vi "LINC Daemon Client.vi"(6 "instance":i32, 7 "timeout ms (1000)":i32=1000, 8 "port config":T1, 9 "port":u16, 10 "address":string, 11 "LINC session":refnum<class "LINC.lvclass">) -> ()   [LabVIEW 2018, in "STEPkgDriver_LINC.lvlib" / "LINC.lvclass"]
uses:
  LINC.lvclass
  STEPkgDriver_LINC.lvlib
  LINC Global Mode.ctl
  LINC Global Config Mode.ctl
  LINC Global Session Mode.ctl
  LINC Global Handshake Mode.ctl
  LINC Handshake Internal.ctl
  LINC Command Origin.ctl
  LINC Handshake.ctl
  LINC Daemon Manager Mode.ctl
  LINC Port Config.ctl
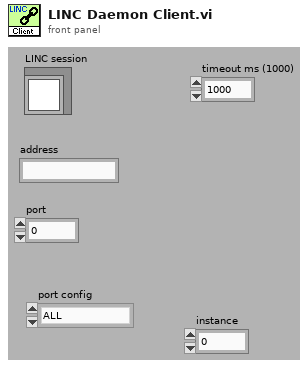
[diagram p1: front panel]
types:
  T1 = typedef "STEPkgDriver_LINC.lvlib/LINC Port Config.ctl" = enum16{"ALL", "CMD_ALL", "TLM_ALL", "TLM_BASIC"}
  T2 = typedef "STEPkgDriver_LINC.lvlib/LINC Global Config Mode.ctl" = enum16{"INIT", "CLEAR", "SET_CMD_CB", "SET_TLM_CB", "SET_CMD_FIELDS", "SET_TLM_FIELDS", "SET_ID", "GET_CONFIG"}
  T3 = typedef "STEPkgDriver_LINC.lvlib/LINC Global Mode.ctl" = enum16{"INIT", "CLEAR", "ADD_PKT_HDR", "ADD_PKT", "GET_PKT_NAMES", "GET_PKT_DESC", "GET_PKT_HDR", "GET_PKT", "SET_PKT", "SET_DATA", "SIM_EN", "SIM_DS"}
  T4 = typedef "STEPkgDriver_LINC.lvlib/LINC Config.ctl" = cluster{"cmd callback":refnum<vi>, "tlm callback":refnum<vi>, "cmd ID bitoffset":i32, "cmd ID bitsize":i32, "cmd IDs":i32[], "tlm ID bitoffset":i32, "tlm ID bitsize":i32, "tlm IDs":i32[], "cmd header fields":i32, "tlm header fields":i32, "tlm header size":i32}
  T5 = typedef "STEPkgDriver_LINC.lvlib/LINC Daemon Manager Mode.ctl" = enum16{"INIT", "CLEAR", "GET"}
  T6 = typedef "STEPkgDriver_LINC.lvlib/LINC Global Session Mode.ctl" = enum16{"INIT", "CLEAR", "ADD_SESSION", "SET_CONNECTION", "SET_LISTENER", "SET_REFERENCE", "GET_SESSION"}
  T7 = cluster{"binary value (F)":bool, "include unit (F)":bool}
  T8 = typedef "STEPkgDriver_LINC.lvlib/LINC Handshake Internal.ctl" = cluster{"error":errorcluster, "command data":string}
  T9 = typedef "STEPkgDriver_LINC.lvlib/LINC Global Handshake Mode.ctl" = enum16{"INIT", "CLEAR", "ADD_COMMAND", "RMV_COMMAND", "CLR_HANDSHAKE", "SET_HANDSHAKE", "GET_HANDSHAKE"}
  T10 = typedef "STEPkgDriver_LINC.lvlib/LINC Handshake.ctl" = cluster{"ORIGIN":T11, "STATUS":bool, "CODE":i32, "TIME_SECONDS":u32, "TIME_MICROSECONDS":u32, "DATA":string}
  T11 = typedef "STEPkgDriver_LINC.lvlib/LINC Command Origin.ctl" = enum8{"RMT", "LCL"}
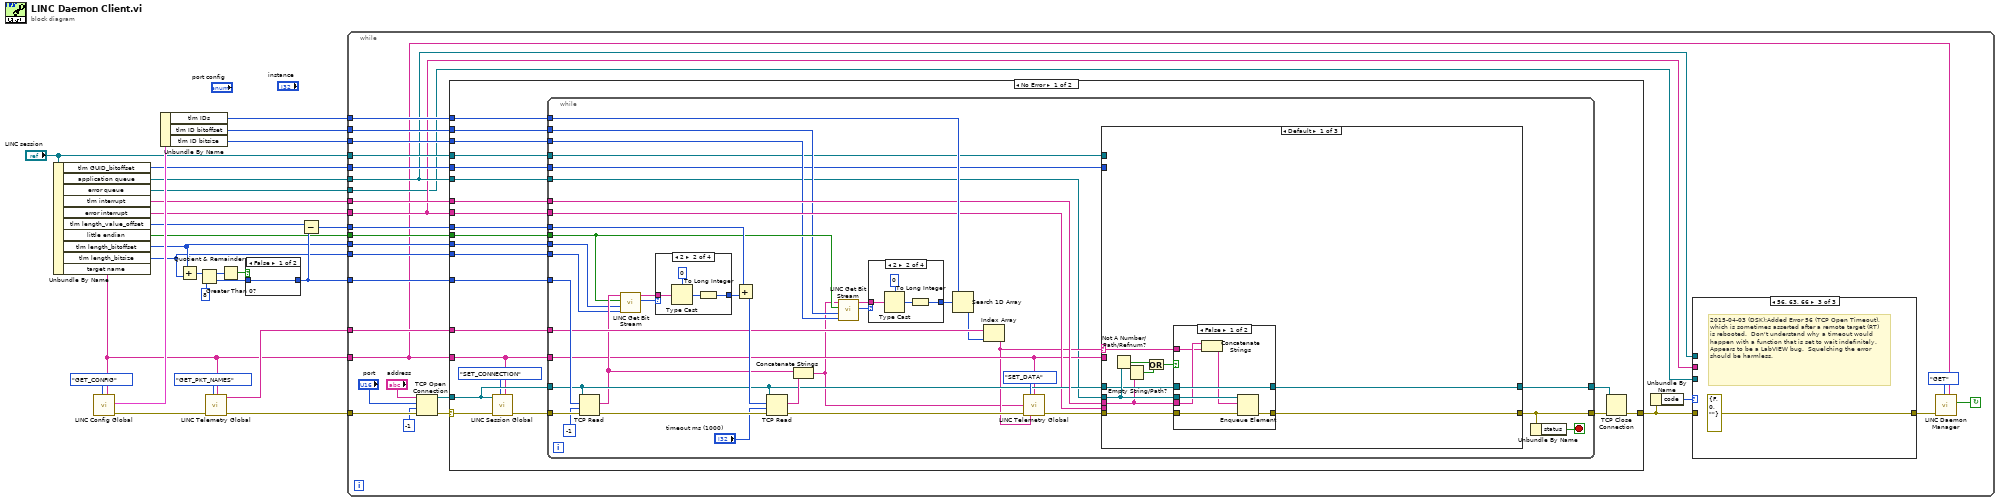
[diagram p0: block diagram]
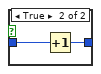
[diagram p2: hidden frame]
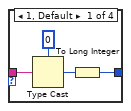
[diagram p3: hidden frame]
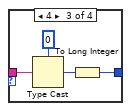
[diagram p4: hidden frame]
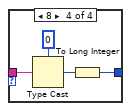
[diagram p5: hidden frame]
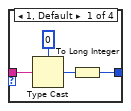
[diagram p6: hidden frame]
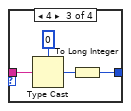
[diagram p7: hidden frame]
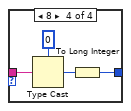
[diagram p8: hidden frame]
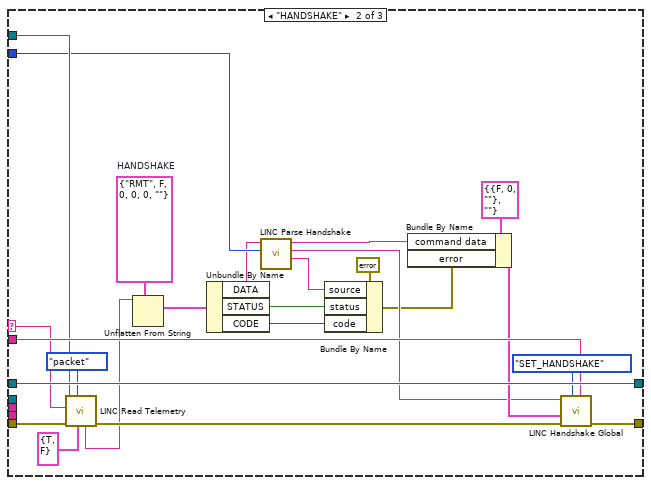
[diagram p10: hidden frame]
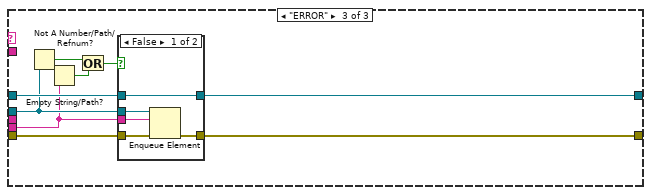
[diagram p11: hidden frame]
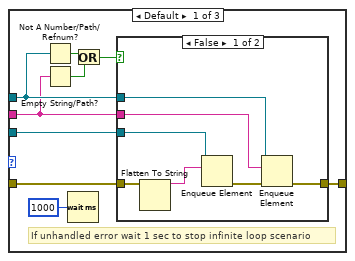
[diagram p14: hidden frame]
diagram:
  n1 = Unbundle By Name("LINC session") -> ("tlm GUID_bitoffset"=w3:i32, "application queue"=w8:refnum<queue>, "error queue"=w1:refnum<queue>, "tlm interrupt"=w9:string, "error interrupt"=w7:string, "tlm length_value_offset"=w10:i32, "little endian"=w6:bool, "tlm length_bitoffset"=w5:i32, "tlm length_bitsize"=w4:i32, "target name"=w11:string)
  n2 = call "LINC Config Global.vi"("target name"=w11, "mode"=LINC_Global_Config_Mode."GET_CONFIG") -> ("error out"=w26:errorcluster, "config out"=w24:T4)  [unwired: 8 in]
  n3 = Unbundle By Name(w24) -> ("tlm IDs"=w23:i32[], "tlm ID bitoffset"=w22:i32, "tlm ID bitsize"=w21:i32)
  n4 = Add(x=w5, y=w4) -> (x+y=w15:i32)
  n5 = Quotient & Remainder(x=w15, y=8) -> (x-y*floor(x/y)=w17:i32, floor(x/y)=w19:i32)
  n6 = call "LINC Telemetry Global.vi"("mode"=LINC_Global_Mode."GET_PKT_NAMES", "target name"=w11, "error in (no error)"=w26) -> ("values out"=w20:string[], "error out"=w25:errorcluster)  [unwired: 8 in, 3 out]
  n7 = Greater Than 0?(x=w17) -> (x > 0?=w18:bool)
  n8 = case shown="False" w18 {
    tunnel: w19 -> [w28 w30]
    tunnel: [w28 w29] -> w13
    frame False {
    }
    frame True {
      n9 = Increment(x=w30) -> (x+1=w29:i32)
    }
  }
  n10 = Subtract(x=w10, y=w13) -> (x-y=w14:i32)
  n11 = while {
    tunnel: w11 -> [w32]
    tunnel: w25 -> [w55]
    tunnel: w23 -> [w54]
    tunnel: w22 -> [w53]
    tunnel: w21 -> [w52]
    tunnel: w20 -> [w51]
    tunnel: w14 -> [w50]
    tunnel: w13 -> [w49]
    tunnel: w9 -> [w48]
    tunnel: w8 -> [w38]
    tunnel: w7 -> [w37]
    tunnel: w6 -> [w45]
    tunnel: w5 -> [w44]
    tunnel: w4 -> [w43]
    tunnel: w3 -> [w42]
    tunnel: "LINC session" -> [w41]
    tunnel: w1 -> [w36]
    stop <- w33 continue-if-true
    n12 = TCP Open Connection(address="address", remote port or service name="port", timeout ms (60000)=-1, error in (no error)=w55) -> (connection ID=w46:refnum<k5>, error out=w31:errorcluster)  [unwired: 1 in]
    n13 = case shown="No Error" w31 {
      selector: w31 -> [w58 w209]
      tunnel: w54 -> [w78 _]
      tunnel: w53 -> [w77 _]
      tunnel: w52 -> [w76 _]
      tunnel: w51 -> [w75 _]
      tunnel: w50 -> [w72 _]
      tunnel: w49 -> [w71 _]
      tunnel: w48 -> [w70 _]
      tunnel: w46 -> [w69 _]
      tunnel: w45 -> [w67 _]
      tunnel: w44 -> [w66 _]
      tunnel: w43 -> [w65 _]
      tunnel: w42 -> [w64 _]
      tunnel: w41 -> [w63 _]
      tunnel: [w62 w209] -> w39
      tunnel: w38 -> [w61 _]
      tunnel: w37 -> [w60 _]
      tunnel: w32 -> [w59 _]
      frame No Error {
        n14 = call "LINC Session Global.vi"("target name"=w59, "mode"=LINC_Global_Session_Mode."SET_CONNECTION", "error in (no error)"=w58, "connection in"=w69) -> ("error out"=w79:errorcluster)  [unwired: 3 in, 4 out]
        n15 = while {
          tunnel: w79 -> [w117]
          tunnel: w69 -> [w101]
          tunnel: [w103] -> w74
          tunnel: [w100] -> w73
          tunnel: w71 -> [w112]
          tunnel: w72 -> [w111]
          tunnel: w76 -> [w88]
          tunnel: w77 -> [w89]
          tunnel: w78 -> [w108]
          tunnel: w75 -> [w109]
          tunnel: w59 -> [w86]
          tunnel: w70 -> [w102]
          tunnel: w61 -> [w81]
          tunnel: w60 -> [w99]
          tunnel: w67 -> [w90]
          tunnel: w66 -> [w94]
          tunnel: w65 -> [w93]
          tunnel: w64 -> [w84]
          tunnel: w63 -> [w82]
          stop <- w115 stop-if-true
          n16 = TCP Read(connection ID=w101, bytes to read=w112, error in (no error)=w117, 9:-1 ("timeout ms (25000)")) -> (data out=w95:string, error out=w114:errorcluster)  [unwired: 2 out]
          n17 = call "LINC Get Bit Stream.vi"("bit size"=w93, "bit offset"=w94, "little endian"=w90, "data in"=w95) -> ("bytes"=w98:i32, "data out"=w97:string)  [unwired: 6 in]
          n18 = case shown="2" w98 {
            tunnel: w97 -> [w137 w141 w145 w149]
            tunnel: [w134 w138 w142 w146] -> w96
            frame 1, Default {
              n19 = Type Cast(type=u8 0, x=w137) -> (*(type *) &x=w135:u8)
              n20 = To Long Integer(number=w135) -> (32bit integer=w134:i32)
            }
            frame 2 {
              n21 = Type Cast(type=u16 0, x=w141) -> (*(type *) &x=w139:u16)
              n22 = To Long Integer(number=w139) -> (32bit integer=w138:i32)
            }
            frame 4 {
              n23 = Type Cast(type=u32 0, x=w145) -> (*(type *) &x=w143:u32)
              n24 = To Long Integer(number=w143) -> (32bit integer=w142:i32)
            }
            frame 8 {
              n25 = Type Cast(type=u64 0, x=w149) -> (*(type *) &x=w147:u64)
              n26 = To Long Integer(number=w147) -> (32bit integer=w146:i32)
            }
          }
          n27 = Add(x=w111, y=w96) -> (x+y=w110:i32)
          n28 = TCP Read(connection ID=w101, bytes to read=w110, error in (no error)=w114, 9:"timeout ms (1000)") -> (data out=w113:string, error out=w105:errorcluster)  [unwired: 2 out]
          n29 = Concatenate Strings(w95, w113) -> (w83:string)
          n30 = call "LINC Get Bit Stream.vi"("bit size"=w88, "bit offset"=w89, "little endian"=w90, "data in"=w83) -> ("bytes"=w91:i32, "data out"=w92:string)  [unwired: 6 in]
          n31 = case shown="2" w91 {
            tunnel: w92 -> [w121 w125 w129 w133]
            tunnel: [w118 w122 w126 w130] -> w87
            frame 1, Default {
              n32 = Type Cast(type=u8 0, x=w121) -> (*(type *) &x=w119:u8)
              n33 = To Long Integer(number=w119) -> (32bit integer=w118:i32)
            }
            frame 2 {
              n34 = Type Cast(type=u16 0, x=w125) -> (*(type *) &x=w123:u16)
              n35 = To Long Integer(number=w123) -> (32bit integer=w122:i32)
            }
            frame 4 {
              n36 = Type Cast(type=u32 0, x=w129) -> (*(type *) &x=w127:u32)
              n37 = To Long Integer(number=w127) -> (32bit integer=w126:i32)
            }
            frame 8 {
              n38 = Type Cast(type=u64 0, x=w133) -> (*(type *) &x=w131:u64)
              n39 = To Long Integer(number=w131) -> (32bit integer=w130:i32)
            }
          }
          n40 = Search 1D Array(1D array=w108, element=w87) -> (index of element=w107:i32)  [unwired: 1 in]
          n41 = Index Array(array=w109, index=w107) -> (element=w85:string)
          n42 = call "LINC Telemetry Global.vi"("mode"=LINC_Global_Mode."SET_DATA", "target name"=w86, "data in"=w83, "error in (no error)"=w105, "packet name"=w85) -> ("error out"=w104:errorcluster)  [unwired: 6 in, 4 out]
          n43 = case shown="Default" w85 {
            selector: w85 -> [w150 w186 _]
            tunnel: w104 -> [w159 w187 w201]
            tunnel: [w158 w190 w200] -> w103
            tunnel: w102 -> [w154 _ _]
            tunnel: w81 -> [w157 _ w195]
            tunnel: w101 -> [w156 w192 w199]
            tunnel: [w155 w192 w198] -> w100
            tunnel: w99 -> [_ _ w194]
            tunnel: w86 -> [_ w189 _]
            tunnel: w84 -> [_ w183 _]
            tunnel: w82 -> [_ w184 _]
            frame Default {
              n44 = Not A Number/Path/Refnum?(number/path/refnum=w157) -> (NaN/Path/Refnum?=w153:bool)
              n45 = Empty String/Path?(string/path=w154) -> (empty?=w152:bool)
              n46 = Or(x=w153, y=w152) -> (x .or. y?=w151:bool)
              n47 = case shown="False" w151 {
                tunnel: w159 -> [w166 w168]
                tunnel: [w165 w168] -> w158
                tunnel: w157 -> [w164 _]
                tunnel: w154 -> [w161 _]
                tunnel: w156 -> [w163 w167]
                tunnel: [w163 w167] -> w155
                tunnel: w150 -> [w160 _]
                frame False {
                  n48 = Concatenate Strings(w161, w160) -> (w162:string)
                  n49 = Enqueue Element(queue=w164, element=w162, error in (no error)=w166) -> (error out=w165:errorcluster)  [unwired: 1 in, 2 out]
                }
                frame True {
                }
              }
            }
            frame "HANDSHAKE" {
              w180 = T10 {"ORIGIN"=enum."RMT", "STATUS"=FALSE, "CODE"=0, "TIME_SECONDS"=0, "TIME_MICROSECONDS"=0, "DATA"=""}  # HANDSHAKE
              n50 = call "LINC Read Telemetry.vi"("options"=T7 {"binary value (F)"=TRUE, "include unit (F)"=FALSE}, "mode (single)"=enum16{"single", "packet", "all"}."packet", "error in (no error)"=w187, "packet name"=w186, "LINC session"=w184) -> ("error out"=w185:errorcluster, "flattened data"=w179:string)  [unwired: 2 in, 3 out]
              n51 = Unflatten From String(type=w180, binary string=w179) -> (value=w178:T10)  [unwired: 3 in, 2 out]
              n52 = Unbundle By Name(w178) -> ("DATA"=w177:string, "STATUS"=w174:bool, "CODE"=w173:i32)
              n53 = call "LINC Parse Handshake.vi"("GUID bitoffset"=w183, "command packet"=w177) -> ("error source"=w169:string, "GUID"=w172:string, "command data"=w170:string)  [unwired: 7 in]
              n54 = Bundle By Name(cluster=errorcluster {"status"=FALSE, "code"=0, "source"=""} ("error out"), "source"=w169, "status"=w174, "code"=w173) -> (w171:errorcluster)
              n55 = Bundle By Name(cluster=T8 {"error"={"status"=FALSE, "code"=0, "source"=""}, "command data"=""} ("handshake in"), "command data"=w170, "error"=w171) -> (w182:T8)
              n56 = call "LINC Handshake Global.vi"("target name"=w189, "mode"=LINC_Global_Handshake_Mode."SET_HANDSHAKE", "error in (no error)"=w185, "handshake in"=w182, "GUID"=w172) -> ("error out"=w190:errorcluster)  [unwired: 3 in, 3 out]
            }
            frame "ERROR" {
              n57 = Not A Number/Path/Refnum?(number/path/refnum=w195) -> (NaN/Path/Refnum?=w197:bool)
              n58 = Empty String/Path?(string/path=w194) -> (empty?=w196:bool)
              n59 = Or(x=w197, y=w196) -> (x .or. y?=w193:bool)
              n60 = case shown="False" w193 {
                tunnel: w201 -> [w206 w208]
                tunnel: [w205 w208] -> w200
                tunnel: w195 -> [w204 _]
                tunnel: w194 -> [w203 _]
                tunnel: w199 -> [w202 w207]
                tunnel: [w202 w207] -> w198
                frame False {
                  n61 = Enqueue Element(queue=w204, element=w203, error in (no error)=w206) -> (error out=w205:errorcluster)  [unwired: 1 in, 2 out]
                }
                frame True {
                }
              }
            }
          }
          n62 = Unbundle By Name(w103) -> ("status"=w115:bool)
        }
        n63 = TCP Close Connection(connection ID=w73, error in (no error)=w74) -> (error out=w62:errorcluster)  [unwired: 1 in, 1 out]
      }
      frame Error {
      }
    }
    n64 = Unbundle By Name(w39) -> ("code"=w40:i32)
    n65 = case shown="56, 63, 66" w40 {
      tunnel: w39 -> [w213 w227 _]
      tunnel: [w212 w227 errorcluster {"status"=FALSE, "code"=0, "source"=""} ("error out")] -> w34
      tunnel: w38 -> [w216 _ _]
      tunnel: w37 -> [w215 _ _]
      tunnel: w36 -> [w211 _ _]
      frame Default {
        # "If unhandled error wait 1 sec to stop infinite loop scenario"
        n66 = Not A Number/Path/Refnum?(number/path/refnum=w216) -> (NaN/Path/Refnum?=w217:bool)
        n67 = Empty String/Path?(string/path=w215) -> (empty?=w218:bool)
        n68 = Wait (ms)(milliseconds to wait=u32 1000) -> ()  [unwired: 1 out]
        n69 = Or(x=w217, y=w218) -> (x .or. y?=w214:bool)
        n70 = case shown="False" w214 {
          tunnel: w216 -> [w225 _]
          tunnel: w215 -> [w224 _]
          tunnel: w213 -> [w222 w226]
          tunnel: [w223 w226] -> w212
          tunnel: w211 -> [w219 _]
          frame False {
            n71 = Flatten To String(anything=w222) -> (data string=w220:string)  [unwired: 3 in, 2 out]
            n72 = Enqueue Element(queue=w219, element=w220) -> (error out=w221:errorcluster)  [unwired: 2 in, 2 out]
            n73 = Enqueue Element(queue=w225, element=w224, error in (no error)=w221) -> (error out=w223:errorcluster)  [unwired: 1 in, 2 out]
          }
          frame True {
          }
        }
      }
      frame 1 {
      }
      frame 56, 63, 66 {
        # "2015-04-03 (DSK):Added Error 56 (TCP Open Timeout), which is sometimes asserted after a remote target (RT) is rebooted.  Don't understand why a timeout would happen with a function that is set to wait indefinitely.  Appears to be a LabVIEW bug.  Squelching the error should be harmless."
      }
    }
    n74 = call "LINC Daemon Manager.vi"("target name"=w32, "mode"=LINC_Daemon_Manager_Mode."GET", "error in (no error)"=w34) -> ("running"=w33:bool)  [unwired: 7 in, 1 out]
  }
